vi "log-all-data.vi"(0 "log-file-byte-stream":refnum<file>, 1 "CSV Data Headings":string, 2 "adam5000:all-data-in":T3, 3 "log-start-time(mS)":u32, 4 "file open?":bool, 5 "error in (no error)":errorcluster, 6 "Log Filepath Selection":T2, 7 "Start Logging":bool, 8 "Enable Log Trigger":bool) -> (10 "appended path for log file":path, 11 "log-elapsed time":dbl format="%.2f", 12 "log-filepath-enable-state":T1(ring), 13 "Start Logging":bool, 14 "log-file-bytestream":refnum<file>, 15 "Logged Data String":string, 17 "log-start-time(mS)":u32, 18 "file open?":bool, 19 "error out":errorcluster)   [LabVIEW 2024]
uses:
  controls/adam-5000-all-chassis-data.ctl
  controls/adam-5000-all-module-datas.ctl
  controls/digital-output-cluster.ctl
  controls/digitial-input-cluster.ctl
  controls/analog-output-cluster.ctl
  controls/analog-input-cluster.ctl
  controls/thermocouple-input-cluster.ctl
  csv-file-logging/filepath-selection.ctl
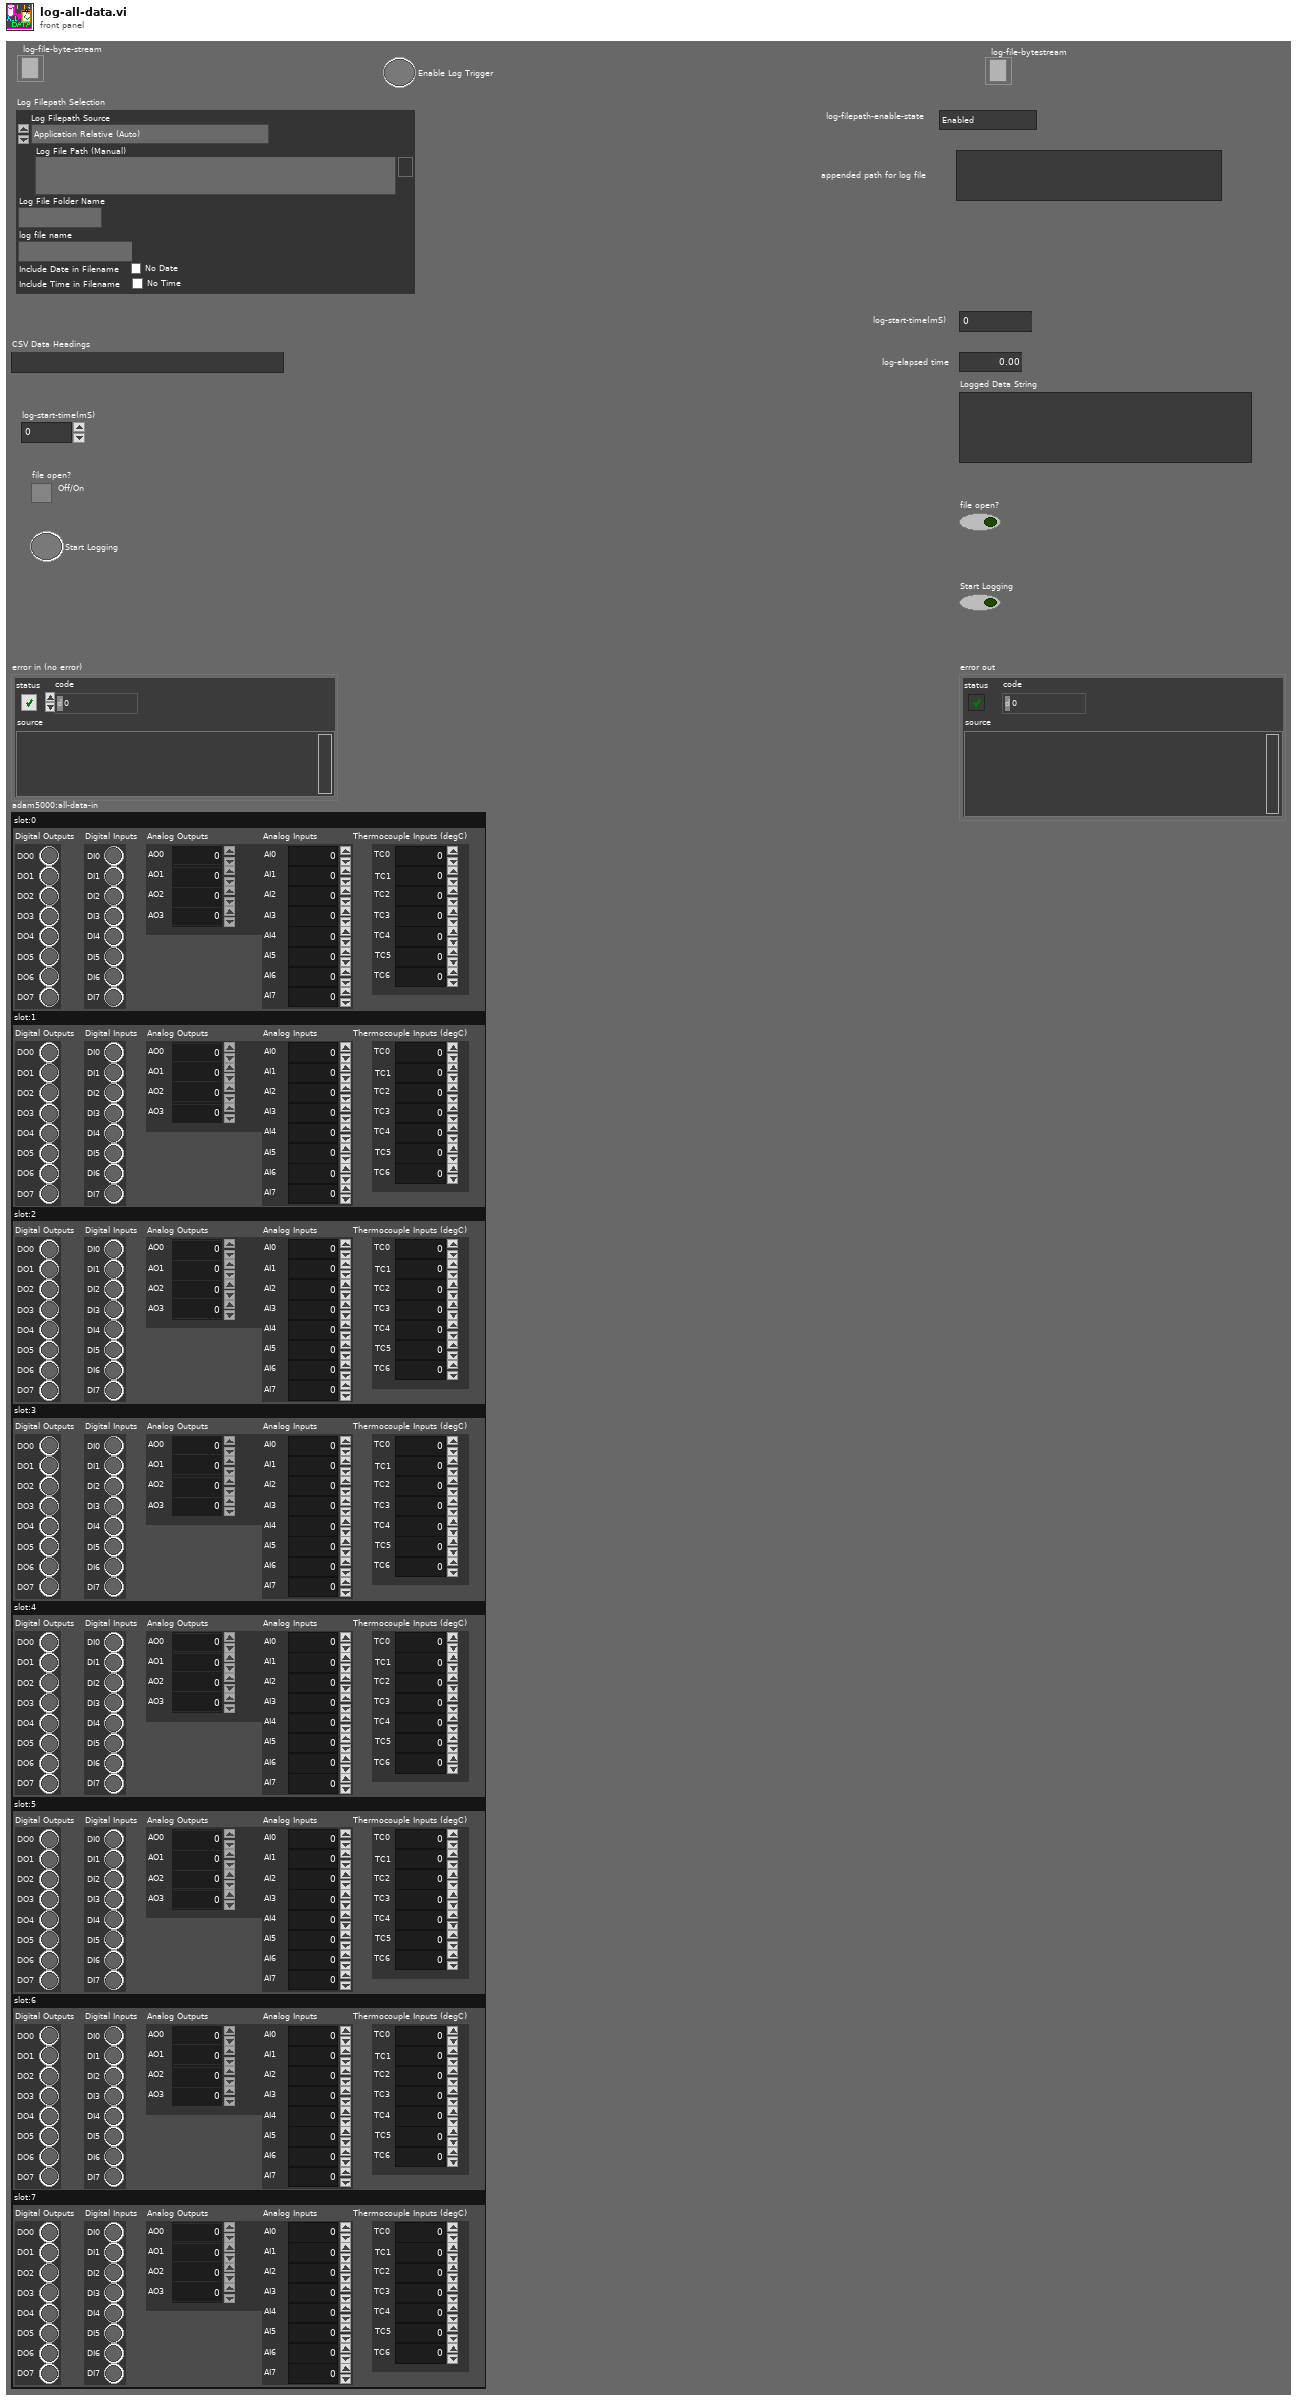
[diagram p1: front panel]
types:
  T1 = enum8{"Enabled", "Disabled", "Disabled and Grayed Out"}
  T2 = typedef "filepath-selection.ctl" = cluster{"Log Filepath Source":enum16{"Application Relative (Auto)", "VI Relative (Auto)", "Complete Path (Manual)"}, "Log File Path (Manual)":path, "Log File Folder Name":string, "log file name":string, "Include Date in Filename":bool, "Include Time in Filename":bool}
  T3 = typedef "adam-5000-all-chassis-data.ctl" = cluster{"slot:0":T4, "slot:1":T4, "slot:2":T4, "slot:3":T4, "slot:4":T4, "slot:5":T4, "slot:6":T4, "slot:7":T4}
  T4 = typedef "adam-5000-all-module-datas.ctl" = cluster{"Digital Outputs":T5, "Digital Inputs":T6, "Analog Outputs":T7, "Analog Inputs":T8, "Thermocouple Inputs (degC)":T9}
  T5 = typedef "digital-output-cluster.ctl" = cluster{"DO0":bool, "DO1":bool, "DO2":bool, "DO3":bool, "DO4":bool, "DO5":bool, "DO6":bool, "DO7":bool}
  T6 = typedef "digitial-input-cluster.ctl" = cluster{"DI0":bool, "DI1":bool, "DI2":bool, "DI3":bool, "DI4":bool, "DI5":bool, "DI6":bool, "DI7":bool}
  T7 = typedef "analog-output-cluster.ctl" = cluster{"AO0":dbl, "AO1":dbl, "AO2":dbl, "AO3":dbl}
  T8 = typedef "analog-input-cluster.ctl" = cluster{"AI0":dbl, "AI1":dbl, "AI2":dbl, "AI3":dbl, "AI4":dbl, "AI5":dbl, "AI6":dbl, "AI7":dbl}
  T9 = typedef "thermocouple-input-cluster.ctl" = cluster{"TC0":dbl, "TC1":dbl, "TC2":dbl, "TC3":dbl, "TC4":dbl, "TC5":dbl, "TC6":dbl}
  T10 = enum16{"open", "replace", "create", "open or create", "replace or create", "replace or create with confirmation"}
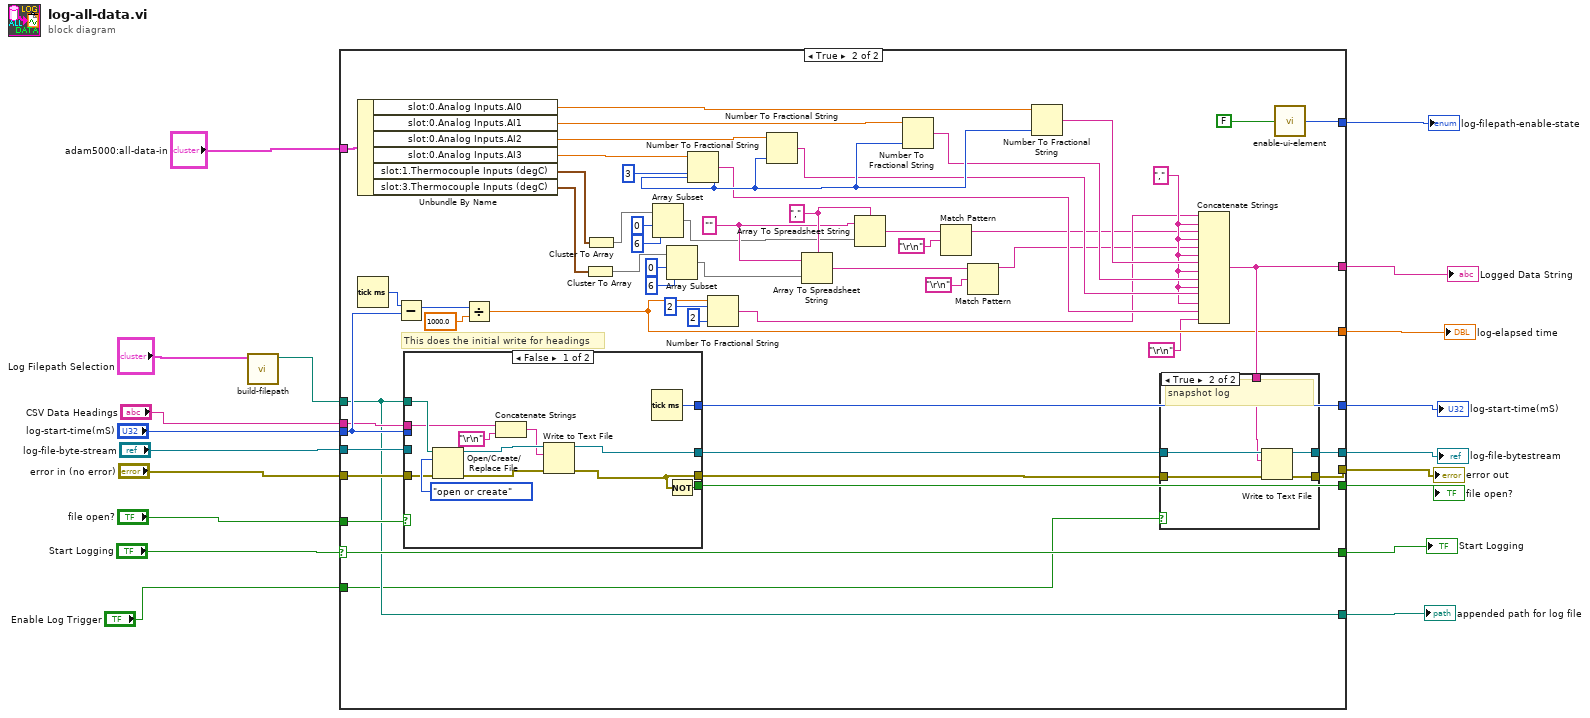
[diagram p0: block diagram]
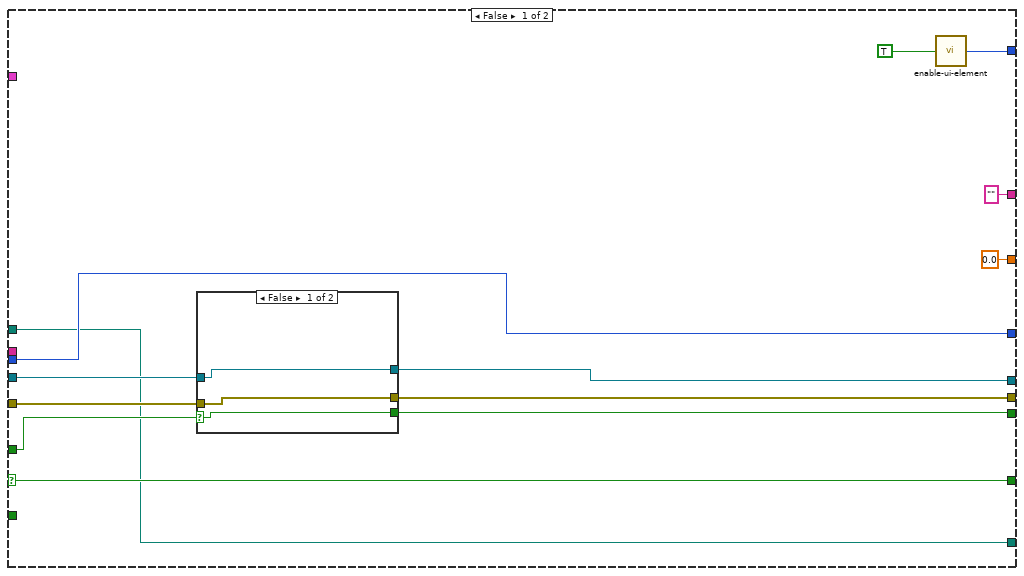
[diagram p2: hidden frame]
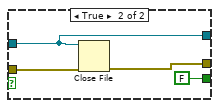
[diagram p3: hidden frame]
diagram:
  n1 = call "build-filepath.vi"("Log Filepath Selection"="Log Filepath Selection") -> ("appended path for log file"=w11:path)  [unwired: 9 in, 1 out]
  n2 = case shown="True" "Start Logging" {
    selector: "Start Logging" -> [w32 w90]
    tunnel: [w32 w90] -> w8
    tunnel: [w23 w91] -> w9
    tunnel: w11 -> [w22 w58]
    tunnel: "adam5000:all-data-in" -> [_ w93]
    tunnel: [w30 w87] -> w13
    tunnel: "file open?" -> [w31 w89]
    tunnel: "error in (no error)" -> [w28 w88]
    tunnel: [w27 w77] -> w15
    tunnel: [w26 w79] -> w16
    tunnel: "log-file-byte-stream" -> [w29 w86]
    tunnel: [w25 w85] -> w18
    tunnel: "log-start-time(mS)" -> [w25 w83]
    tunnel: "CSV Data Headings" -> [_ w81]
    tunnel: ["" w73] -> w4
    tunnel: [0.0 w66] -> w3
    tunnel: [w22 w58] -> w2
    tunnel: "Enable Log Trigger" -> [_ w40]
    frame False {
      n3 = case shown="False" w31 {
        selector: w31 -> [w33 _]
        tunnel: [w33 FALSE] -> w30
        tunnel: w29 -> [w35 w36]
        tunnel: w28 -> [w34 w38]
        tunnel: [w34 w37] -> w27
        tunnel: [w35 w36] -> w26
        frame False {
        }
        frame True {
          n4 = Close File(refnum=w36, error in=w38) -> (error out=w37:errorcluster)  [unwired: 1 out]
        }
      }
      n5 = call "enable-ui-element.vi"("Enable UI Element"=TRUE) -> ("UI Element State"=w23:T1)  [unwired: 8 in]
    }
    frame True {
      w56 = "" ("format string")
      w64 = "," ("delimiter (Tab)")
      w59 = "," ("string")
      w67 = i16 3 ("precision (6)")
      # "This does the initial write for headings"
      n6 = Unbundle By Name(w93) -> ("slot:0.Analog Inputs.AI0"=w76:dbl, "slot:0.Analog Inputs.AI1"=w72:dbl, "slot:0.Analog Inputs.AI2"=w71:dbl, "slot:0.Analog Inputs.AI3"=w75:dbl, "slot:1.Thermocouple Inputs (degC)"=w69:T9, "slot:3.Thermocouple Inputs (degC)"=w68:T9)
      n7 = Tick Count (ms)() -> (millisecond timer value=w84:u32)
      n8 = Subtract(x=w84, y=w83) -> (x-y=w82:u32)
      n9 = case shown="False" w89 {
        selector: w89 -> [_ w116]
        tunnel: w58 -> [w111 _]
        tunnel: w88 -> [w110 w115]
        tunnel: [w105 w115] -> w78
        tunnel: [w109 w116] -> w87
        tunnel: [w104 w113] -> w80
        tunnel: w86 -> [_ w113]
        tunnel: [w108 w114] -> w85
        tunnel: w83 -> [_ w114]
        tunnel: w81 -> [w102 _]
        frame False {
          n10 = Open/Create/Replace File(file path (use dialog)=w111, error in=w110, operation (0:open)=T10."open or create") -> (refnum out=w107:refnum<file>, error out=w106:errorcluster)  [unwired: 3 in, 1 out]
          n11 = Concatenate Strings(w102, "\r\n") -> (w101:string)
          n12 = Write to Text File(file (use dialog)=w107, text=w101, error in=w106) -> (refnum out=w104:refnum<file>, error out=w105:errorcluster)  [unwired: 1 in, 1 out]
          n13 = Tick Count (ms)() -> (millisecond timer value=w108:u32)
          n14 = Not(x=w105) -> (.not. x?=w109:bool)
        }
        frame True {
        }
      }
      n15 = Divide(x=w82, y=1000.0) -> (x/y=w66:dbl)
      n16 = Cluster To Array(cluster=w68) -> (array=w43:dbl[])
      n17 = Cluster To Array(cluster=w69) -> (array=w49:dbl[])
      n18 = Array Subset(array=w49, index=0, length=6) -> (w46:dbl[])
      n19 = Array Subset(array=w43, index=0, length=6) -> (w42:dbl[])
      n20 = Number To Fractional String(number=w75, precision (6)=w67) -> (F-format string=w63:string)  [unwired: 2 in]
      n21 = Number To Fractional String(number=w66, width (-)=i16 2, precision (6)=i16 2) -> (F-format string=w57:string)  [unwired: 1 in]
      n22 = Number To Fractional String(number=w71, precision (6)=w67) -> (F-format string=w62:string)  [unwired: 2 in]
      n23 = Array To Spreadsheet String(delimiter (Tab)=w64, array=w42, 3:w56) -> (spreadsheet string=w52:string)
      n24 = Array To Spreadsheet String(delimiter (Tab)=w64, array=w46, 3:w56) -> (spreadsheet string=w55:string)
      n25 = Number To Fractional String(number=w72, precision (6)=w67) -> (F-format string=w61:string)  [unwired: 2 in]
      n26 = Match Pattern(string=w55, regular expression="\r\n") -> (before substring=w54:string)  [unwired: 1 in, 3 out]
      n27 = Match Pattern(string=w52, regular expression="\r\n") -> (before substring=w50:string)  [unwired: 1 in, 3 out]
      n28 = Number To Fractional String(number=w76, precision (6)=w67) -> (F-format string=w60:string)  [unwired: 2 in]
      n29 = Concatenate Strings(w57, w59, w54, w59, w50, w59, w60, w59, w61, w59, w62, w59, w63, "\r\n") -> (w73:string)
      n30 = case shown="True" w40 {
        tunnel: w80 -> [w95 w100]
        tunnel: [w95 w99] -> w79
        tunnel: w78 -> [w94 w98]
        tunnel: [w94 w97] -> w77
        tunnel: w73 -> [_ w96]
        frame False {
        }
        frame True {
          # "snapshot log"
          n31 = Write to Text File(file (use dialog)=w100, text=w96, error in=w98) -> (refnum out=w99:refnum<file>, error out=w97:errorcluster)  [unwired: 1 in, 1 out]
        }
      }
      n32 = call "enable-ui-element.vi"("Enable UI Element"=FALSE) -> ("UI Element State"=w91:T1)  [unwired: 8 in]
    }
  }
  "log-start-time(mS)" <- w18
  "log-file-bytestream" <- w16
  "error out" <- w15
  "file open?" <- w13
  "appended path for log file" <- w2
  "log-filepath-enable-state" <- w9
  "Start Logging" <- w8
  "Logged Data String" <- w4
  "log-elapsed time" <- w3
